vi "json settings file_WS.vi"() -> ()   [LabVIEW 2018]
uses:
  DAQ_inputs/AI channel settings.ctl
  <vilib>/addons/_JKI.lib/Serialization/JSON/JKI JSON Serialization.lvlib
panel:
  in  "DAQmx Physical Channel":tag
  in  "save changes":bool
  in  "Exit":bool
  in  "AI channel setting":T1={"device name"="Dev1", "physical channel"=[], "channel name"=[], "maximum value"=[], "minimum value"=[], "units"=10348} {"units" items=["Volts"=10348, "From TEDS"=12516, "From Custom Scale"=10065]}
  # "DAQmx physical channel control values are not compatible with json.\nSelect the channel, copy and past it under physical channel array.\nIt gets converted back to physical channel control in the channel setting vi."
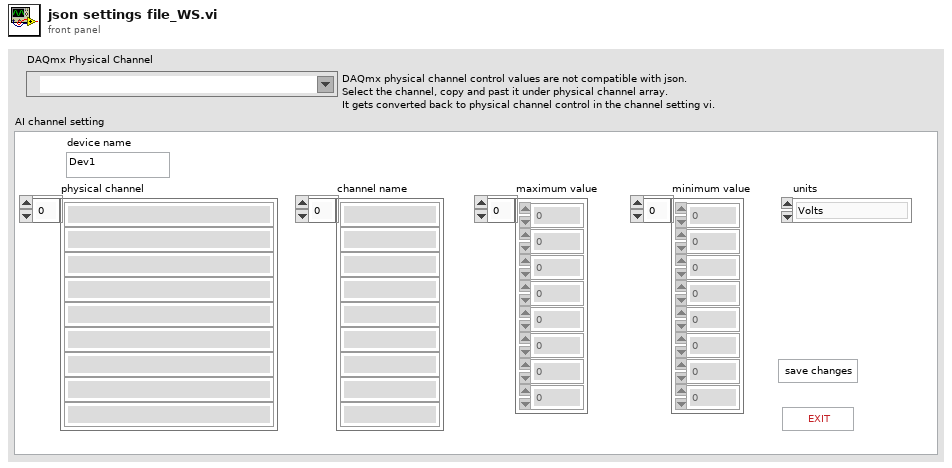
[diagram p1: front panel]
types:
  T1 = typedef "AI channel settings.ctl" = cluster{"device name":string, "physical channel":string[], "channel name":string[], "maximum value":dbl[], "minimum value":dbl[], "units":i32}
  T2 = cluster{"appended path":path, "AI channel settings":T1}
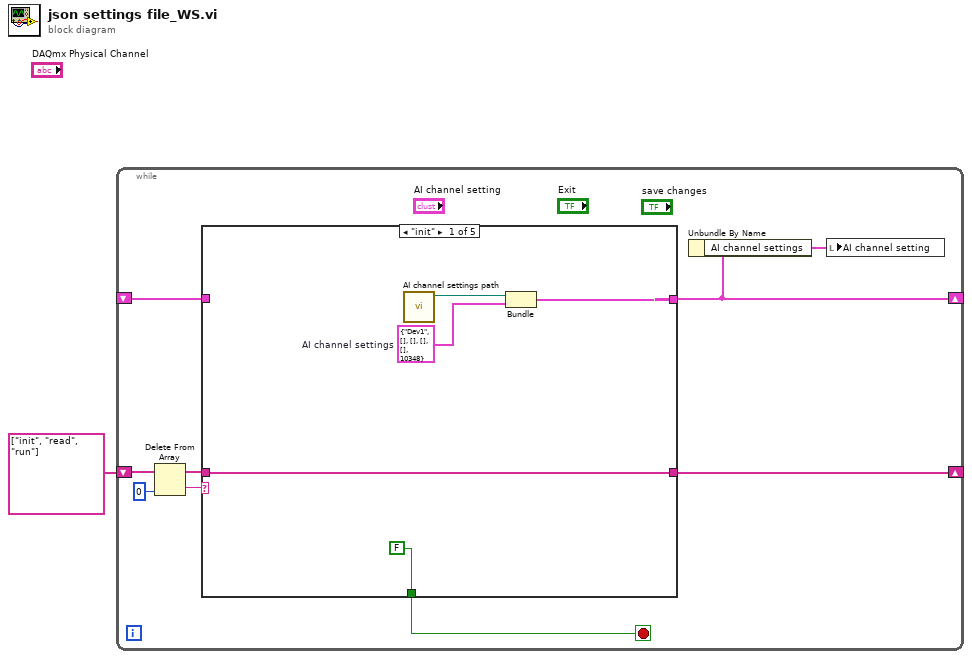
[diagram p0: block diagram]
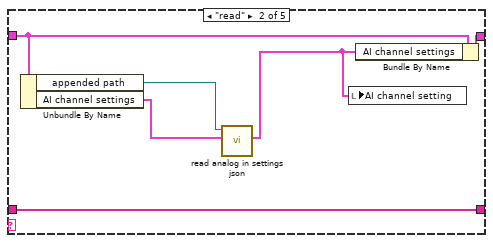
[diagram p2: hidden frame]
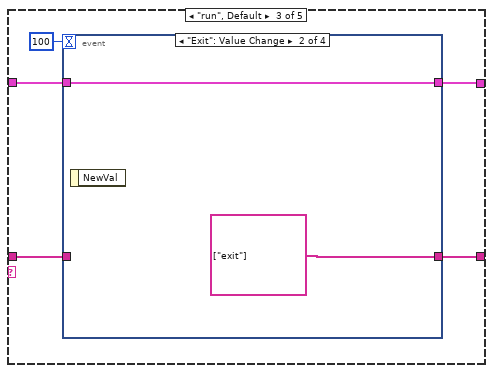
[diagram p3: hidden frame]
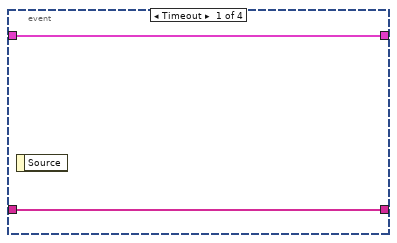
[diagram p4: hidden frame]
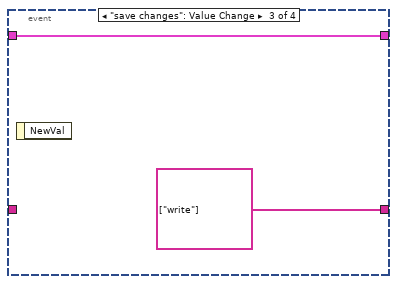
[diagram p5: hidden frame]
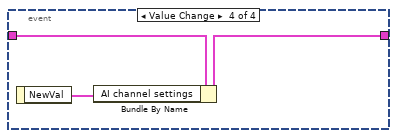
[diagram p6: hidden frame]
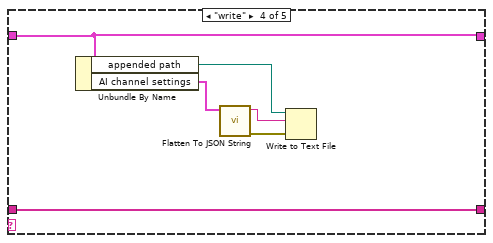
[diagram p7: hidden frame]
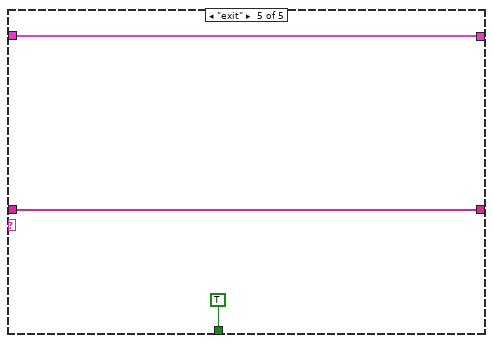
[diagram p8: hidden frame]
diagram:
  n1 = while {
    shift-right: [w10] -> _
    shift-left: string[] ["init", "read", "run"] -> [w4]
    shift-right: [w3] -> _
    shift-left: _ -> [w8]
    stop <- w9 stop-if-true
    n2 = Delete From Array(array=w4, index=0) -> (deleted portion=w5:string, array with subset deleted=w6:string[])  [unwired: 1 in]
    n3 = case shown="\"init\"" w5 {
      tunnel: w6 -> [w15 w21 w26 w41 w44]
      tunnel: [w15 w21 w25 w41 w44] -> w10
      tunnel: [FALSE _ _ _ TRUE] -> w9
      tunnel: [w11 w18 w23 w38 w42] -> w3
      tunnel: w8 -> [_ w20 w24 w38 w42]
      frame "init" {
        w12 = T1 {"device name"="Dev1", "physical channel"=[], "channel name"=[], "maximum value"=[], "minimum value"=[], "units"=10348}  # AI channel settings
        n4 = call "AI channel settings path.vi"() -> ("appended path"=w13:path)  [unwired: 11 in]
        n5 = Bundle("appended path"=w13, "AI channel settings"=w12) -> (w11:T2)  [unwired: 1 in]
      }
      frame "read" {
        n6 = Unbundle By Name(w20) -> ("appended path"=w19:path, "AI channel settings"=w17:T1)
        n7 = call "read analog in settings json.vi"("AI channel type"=w17, "appended path"=w19) -> ("AI channel settings out"=w16:T1)  [unwired: 9 in]
        n8 = local write "AI channel setting"(w16) -> ()
        n9 = Bundle By Name(cluster=w20, "AI channel settings"=w16) -> (w18:T2)
      }
      frame "run", Default {
        n10 = event shown="[1] \"Exit\": Value Change" {
          selector: _ -> [_ _ _ _]
          dyn-events: _ -> [_ _ _ _]
          timeout: 100 -> [_ _ _ _]
          tunnel: [w28 string[] ["exit"] string[] ["write"] _] -> w25
          tunnel: w26 -> [w28 _ _ _]
          tunnel: w24 -> [w27 w29 w31 w35]
          tunnel: [w27 w29 w31 w34] -> w23
          event Timeout {
            n11 = event-data() -> ()  [unwired: 1 in, 1 out]
          }
          event "Exit": Value Change {
            n12 = event-data() -> ()  [unwired: 1 in, 1 out]
          }
          event "save changes": Value Change {
            n13 = event-data() -> ()  [unwired: 1 in, 1 out]
          }
          event Value Change {
            n14 = event-data() -> ("NewVal"=w33:T1)  [unwired: 1 in]
            n15 = Bundle By Name(cluster=w35, "AI channel settings"=w33) -> (w34:T2)
          }
        }
      }
      frame "write" {
        n16 = Unbundle By Name(w38) -> ("appended path"=w36:path, "AI channel settings"=w37:T1)
        n17 = call <vilib>:"Flatten To JSON String.vi"("Variant"=w37) -> ("error out"=w39:errorcluster, "JSON String"=w40:string)  [unwired: 9 in]
        n18 = Write to Text File(file (use dialog)=w36, text=w40, error in=w39) -> ()  [unwired: 1 in, 3 out]
      }
      frame "exit" {
      }
    }
    n19 = Unbundle By Name(w3) -> ("AI channel settings"=w2:T1)
    n20 = local write "AI channel setting"(w2) -> ()
  }
